vi "sync.vi"() -> ()   [LabVIEW 2009]
uses:
  <vilib>/Analysis/NI_AALBase.lvlib
panel:
  out "歪み率":dbl
  out "XYグラフ":cluster{dbl[], dbl[]}(graph)
  in  "位相":dbl
  in  "Q":dbl
  out "送信波":cluster{dbl[], dbl[]}(graph)
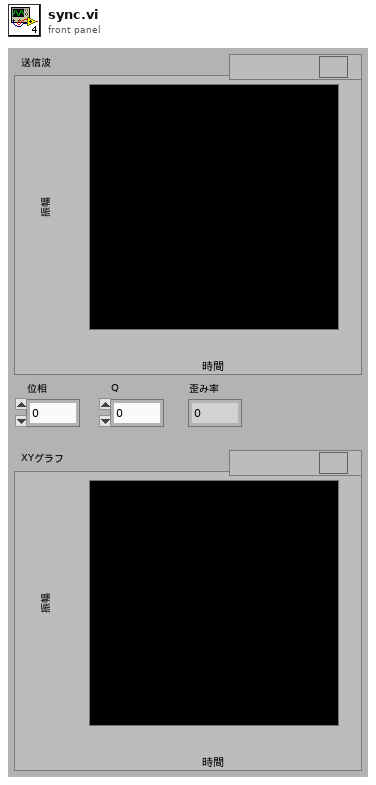
[diagram p1: front panel]
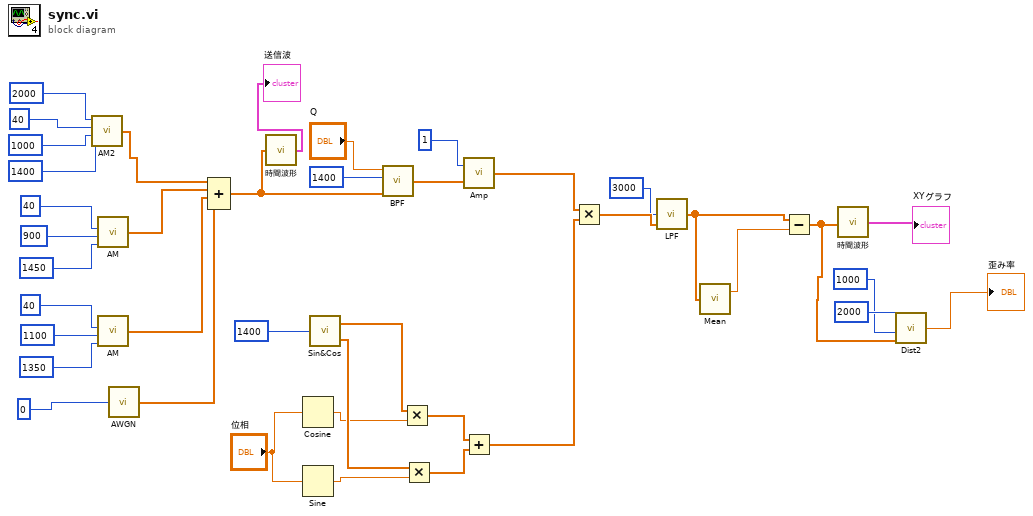
[diagram p0: block diagram]
diagram:
  n1 = call "AM2.vi"("搬送波周波数 [kHz]"=1400, "変調周波数1 [Hz]"=1000, "変調度 [%]"=40, "変調周波数2 [Hz]"=2000) -> ("変調波"=w5:dbl[])  [unwired: 2 in]
  n2 = call "AM.vi"("変調度 [%]"=40, "変調周波数 [Hz]"=900, "搬送波周波数 [kHz]"=1450) -> ("変調波"=w34:dbl[])  [unwired: 2 in]
  n3 = call "AM.vi"("変調度 [%]"=40, "変調周波数 [Hz]"=1100, "搬送波周波数 [kHz]"=1350) -> ("変調波"=w33:dbl[])  [unwired: 2 in]
  n4 = call "AWGN.vi"("振幅値"=0) -> ("出力"=w32:dbl[])
  n5 = Compound Arithmetic op=ADD(w5, w34, w33, w32) -> (w29:dbl[])
  n6 = call "時間波形.vi"("入力"=w29) -> ("時間波形"=→"送信波":cluster{dbl[], dbl[]})
  n7 = Cosine(x="位相") -> (cos(x)=w12:dbl)
  n8 = Sine(x="位相") -> (sin(x)=w10:dbl)
  n9 = call "Sin&Cos.vi"("周波数[kHz]"=1400) -> ("sin"=w19:dbl[], "cos"=w18:dbl[])
  n10 = call "BPF.vi"("X"=w29, "中心周波数 [kHz]"=1400, "Q"="Q") -> ("BPF出力"=w27:dbl[])  [unwired: 1 in]
  n11 = Multiply(x=w19, y=w12) -> (x*y=w17:dbl[])
  n12 = Multiply(x=w18, y=w10) -> (x*y=w16:dbl[])
  n13 = call "Amp.vi"("入力"=w27, "増幅率"=1) -> ("出力"=w24:dbl[])
  n14 = Add(x=w17, y=w16) -> (x+y=w15:dbl[])
  n15 = Multiply(x=w24, y=w15) -> (x*y=w23:dbl[])
  n16 = call "LPF.vi"("入力"=w23, "カットオフ周波数 [Hz]"=3000) -> ("LPF出力"=w13:dbl[])  [unwired: 1 in]
  n17 = call <vilib>:"Mean.vi"("X"=w13) -> ("mean"=w14:dbl)  [unwired: 1 out]
  n18 = Subtract(x=w13, y=w14) -> (x-y=w2:dbl[])
  n19 = call "時間波形.vi"("入力"=w2) -> ("時間波形"=→"XYグラフ":cluster{dbl[], dbl[]})
  n20 = call "Dist2.vi"("入力"=w2, "基本周波数1 [Hz]"=1000, "基本周波数2 [Hz]"=2000) -> ("ひずみ率"=→"歪み率":dbl)  [unwired: 1 in]
